vi "Calculator-setup.vi"(11 "test case ID":string) -> (0 "error out":errorcluster, 1 "Operation":T1, 2 "b":dbl, 3 "a":dbl)   [LabVIEW 2015]
doc: "The setup VI should be executed before the VI under test in the harness VI. In this VI you can prepare the environment and the inputs of the VI under test.\n\nSee the Help Document for more information. (<b>Help</b> > <b>IncQuery Labs</b> > <b>InstaCoverage</b> > <b>InstaCoverage Help...</b>)"
uses:
  Operation.ctl
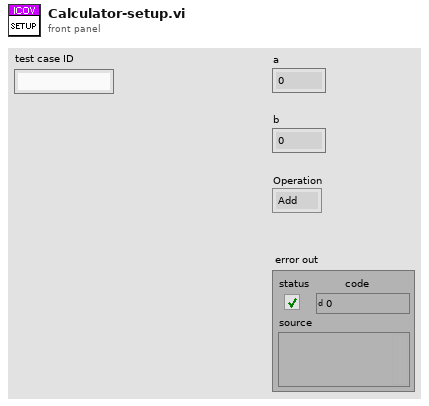
[diagram p1: front panel]
types:
  T1 = typedef "Operation.ctl" = enum16{"Add", "Subtract", "Multiply", "Divide"}
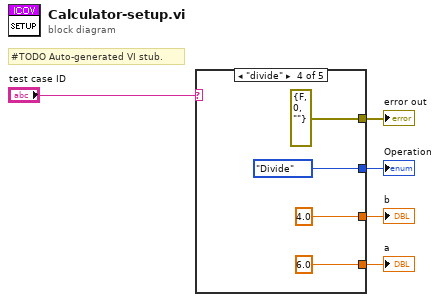
[diagram p0: block diagram]
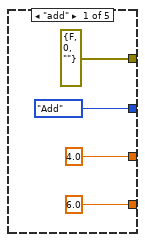
[diagram p2: hidden frame]
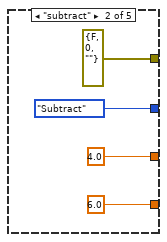
[diagram p3: hidden frame]
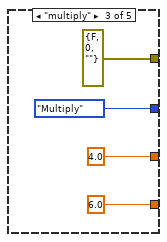
[diagram p4: hidden frame]
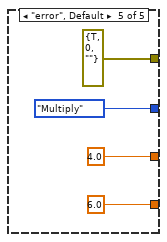
[diagram p5: hidden frame]
diagram:
  # "#TODO Auto-generated VI stub."
  n1 = case shown="\"divide\"" "test case ID" {
    tunnel: [6.0 6.0 6.0 6.0 6.0] -> w4
    tunnel: [4.0 4.0 4.0 4.0 4.0] -> w3
    tunnel: [Operation."Add" ("Operation 2") Operation."Subtract" ("Operation 2") Operation."Multiply" ("Operation 2") Operation."Divide" ("Operation 2") Operation."Multiply" ("Operation 2")] -> w2
    tunnel: [errorcluster {"status"=FALSE, "code"=0, "source"=""} ("error out") errorcluster {"status"=FALSE, "code"=0, "source"=""} ("error out") errorcluster {"status"=FALSE, "code"=0, "source"=""} ("error out") errorcluster {"status"=FALSE, "code"=0, "source"=""} ("error out") errorcluster {"status"=TRUE, "code"=0, "source"=""} ("error out")] -> w1
    frame "add" {
    }
    frame "subtract" {
    }
    frame "multiply" {
    }
    frame "divide" {
    }
    frame "error", Default {
    }
  }
  "a" <- w4
  "b" <- w3
  "Operation" <- w2
  "error out" <- w1
